vi "LVClass_CameraSet Get CameraSpecification.vi"(0 "CameraSet in":refnum<class "CameraSet.lvclass">, 11 "error in (no error)":errorcluster) -> (4 "CameraSet out":refnum<class "CameraSet.lvclass">, 6 "Camera Config":T1, 15 "error out":errorcluster)   [LabVIEW 2020, in "CameraSet.lvclass"]
doc: "Camera specifications getter.\n\n<B>camera_setIn</B> : CameraSet object.\n<B>camera_setOut</B> : CameraSet object.\n<B>driver_name</B> : Camera driver name.\n<B>camera_name</B> : Camera pretty name.\n<B>camera_serial_number</B> : Camera serial number.\n<B>width</B> : Sensor width (pixels).\n<B>height</B> : Sensor height (pixels).\n<B>pixels_stepx</B> : Pixel width (um).\n<B>pixels_stepy</B> : Pixel height (um).\n<B>bits_depth</B> : Image dynamic (number of bytes : 1 for 8 bits, 2 for 16 bits ...).\n<B>is_signed</B> : Indicates if image data is signed.\n<B>max_level</B> : Sensor saturation level (grey level).\n<B>max_frame_rate</B> : Camera maximum framerate (image / s).\n<B>roi_width</B> : Region of interest width.\n<B>roi_height</B> : Region of interest height.\n<B>roi_offsetx</B> : Region of interest top-left corner x coordinate (relative to sensor width).\n<B>roi_offsety</B> : Region of interest top-left corner y coordinate (relative to sensor height)."
uses:
  CameraSet.lvclass
  CameraSpecifications.ctl
  General dimensions definition.ctl
  Point2D.ctl
  Point2Df.ctl
  Data alignment enum.ctl
  CameraSet.lvclass/CameraSet.ctl
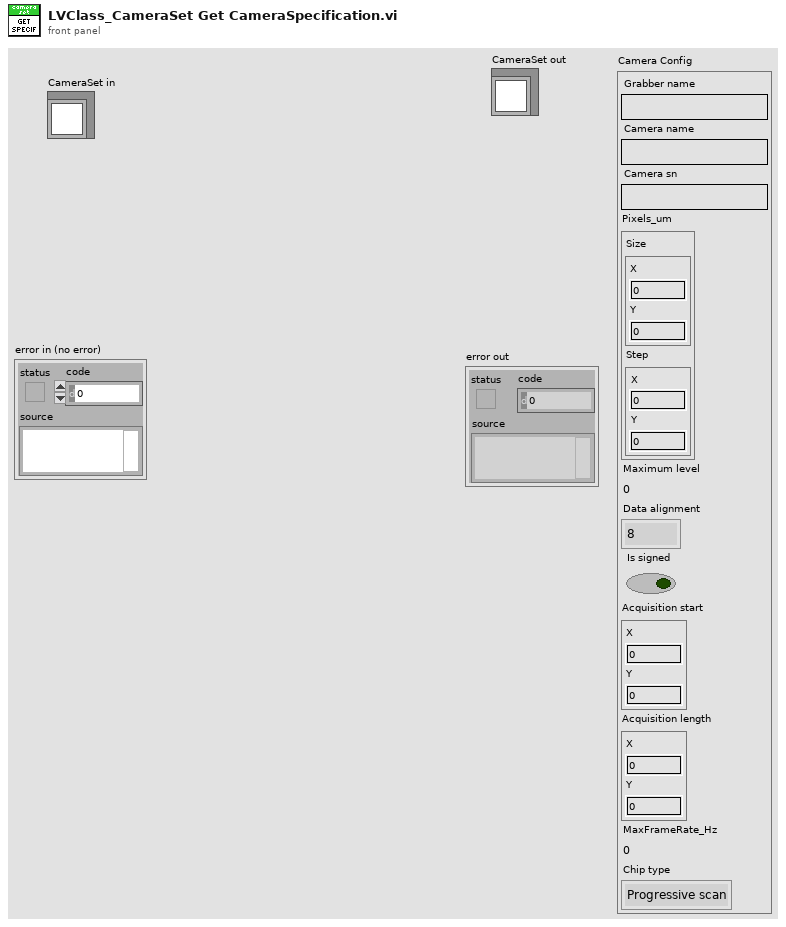
[diagram p1: front panel]
types:
  T1 = typedef "CameraSpecifications.ctl" = cluster{"Grabber name":string, "Camera name":string, "Camera sn":string, "Pixels_um":T2, "Maximum level":u32, "Data alignment":T5, "Is signed":bool, "Acquisition start":T3, "Acquisition length":T3, "MaxFrameRate_Hz":sgl, "Chip type":enum16{"Progressive scan", "Frame transfert"}}
  T2 = typedef "General dimensions definition.ctl" = cluster{"Size":T3, "Step":T4}
  T3 = typedef "Point2D.ctl" = cluster{"X":u32, "Y":u32}
  T4 = typedef "Point2Df.ctl" = cluster{"X":sgl, "Y":sgl}
  T5 = typedef "Data alignment enum.ctl" = enum16{"8", "16", "32"}
  T6 = typedef "ClassID.ctl" = i64
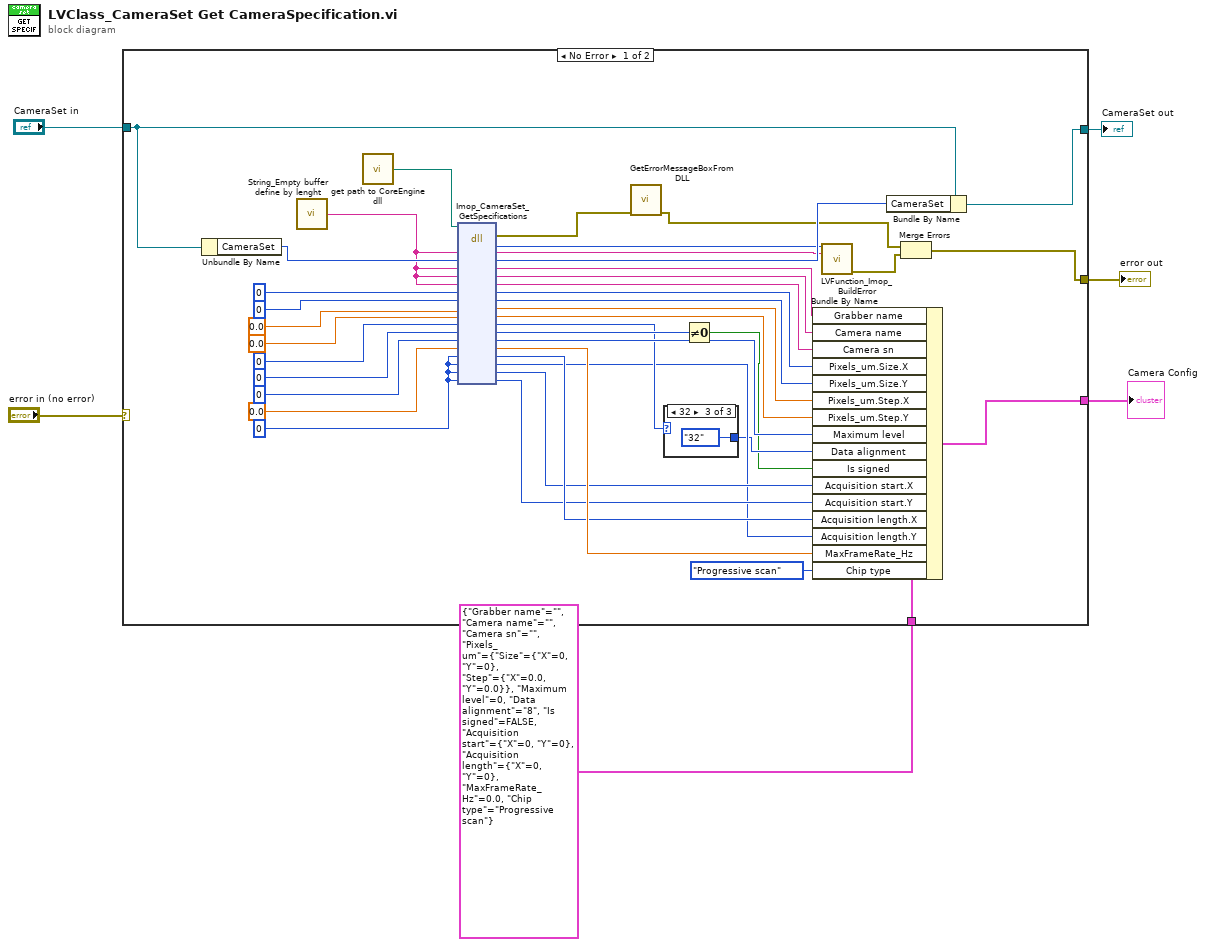
[diagram p0: block diagram]
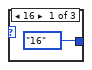
[diagram p2: hidden frame]
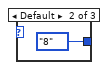
[diagram p3: hidden frame]
diagram:
  n1 = case shown="No Error" "error in (no error)" {
    selector: "error in (no error)" -> [_ w51]
    tunnel: "CameraSet in" -> [w17 w52]
    tunnel: [w44 w52] -> w4
    tunnel: [w13 w51] -> w3
    tunnel: T1 {"Grabber name"="", "Camera name"="", "Camera sn"="", "Pixels_um"={"Size"={"X"=0, "Y"=0}, "Step"={"X"=0.0, "Y"=0.0}}, "Maximum level"=0, "Data alignment"=enum."8", "Is signed"=FALSE, "Acquisition start"={"X"=0, "Y"=0}, "Acquisition length"={"X"=0, "Y"=0}, "MaxFrameRate_Hz"=0.0, "Chip type"=enum."Progressive scan"} ("Camera Config 2") -> [w43 _]
    tunnel: [w37 _] -> w1
    frame No Error {
      w10 = 0 ("roi_offetx")
      n2 = Unbundle By Name(w17) -> ("CameraSet"=w16:T6)
      n3 = call "String_Empty buffer define by lenght.vi"() -> ("Empty buffer"=w8:string)  [unwired: 1 in]
      n4 = call "get path to CoreEngine dll.vi"() -> ("path to c_interface_vc100.dll"=w23:path)  [unwired: 12 in, 3 out]
      n5 = dll-call lib="D:/soft/HASO_v3/SVN_trunk/ImOpCoreEngine4_LV2011/DLLs/c_interface_vc100.dll" fn="Imop_CameraSet_GetSpecifications"(path in=w23, "message"=w8, "objet"=w16, "driver_name"=w8, "camera_name"=w8, "camera_serial_number"=w8, "width"=u32 0, "height"=u32 0, "pixels_stepx"=sgl 0.0, "pixels_stepy"=sgl 0.0, "nb_bits"=u8 0, "is_signed"=u8 0, "max_level"=u64 0, "max_frame_rate"=sgl 0.0, "roi_width"=w10, "roi_height"=w10, "roi_offetx"=w10, "roi_offsety"=w10) -> (error out=w21:errorcluster, "return type"=w45:i32, "message"=w46:string, "objet"=w47:i64, "driver_name"=w36:string, "camera_name"=w35:string, "camera_serial_number"=w34:string, "width"=w33:i32, "height"=w32:i32, "pixels_stepx"=w31:sgl, "pixels_stepy"=w30:sgl, "nb_bits"=w20:u8, "is_signed"=w29:u8, "max_level"=w28:u64, "max_frame_rate"=w27:sgl, "roi_width"=w26:u32, "roi_height"=w19:u32, "roi_offetx"=w25:i32, "roi_offsety"=w24:i32)  [unwired: 2 in, 1 out]
      n6 = call "GetErrorMessageBoxFromDLL.vi"("error IN"=w21) -> ("error OUT"=w14:errorcluster)  [unwired: 10 in]
      n7 = case shown="32" w20 {
        tunnel: [Data_alignment_enum."16" ("Data alignment") Data_alignment_enum."8" ("Data alignment") Data_alignment_enum."32" ("Data alignment")] -> w18
        frame 16 {
        }
        frame Default {
        }
        frame 32 {
        }
      }
      n8 = Not Equal To 0?(x=w29) -> (x != 0?=w11:bool)
      n9 = Bundle By Name(cluster=w43, "Grabber name"=w36, "Camera name"=w35, "Camera sn"=w34, "Pixels_um.Size.X"=w33, "Pixels_um.Size.Y"=w32, "Pixels_um.Step.X"=w31, "Pixels_um.Step.Y"=w30, "Maximum level"=w28, "Data alignment"=w18, "Is signed"=w11, "Acquisition start.X"=w25, "Acquisition start.Y"=w24, "Acquisition length.X"=w26, "Acquisition length.Y"=w19, "MaxFrameRate_Hz"=w27, "Chip type"=enum16{"Progressive scan", "Frame transfert"}."Progressive scan") -> (w37:T1)
      n10 = call "LVFunction_Imop_BuildError.vi"("code"=w45, "String to Prepend to source (\"\")"=w46) -> ("error out"=w15:errorcluster)  [unwired: 13 in]
      n11 = Bundle By Name(cluster=w17, "CameraSet"=w47) -> (w44:refnum<class "CameraSet.lvclass">)
      n12 = Merge Errors(w14, w15) -> (w13:errorcluster)
    }
    frame Error {
    }
  }
  "CameraSet out" <- w4
  "error out" <- w3
  "Camera Config" <- w1
